vi "niRFUtil MASMT Get 1D CSG Type.vi"(1 "1D CSG Array in":csg[](array[numeric])) -> (0 "1D CSG Array out":csg[](array[numeric]))   [LabVIEW 2016, in "niRFUtil.lvlib"]
uses:
  niRFUtil.lvlib
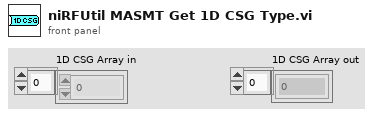
[diagram p1: front panel]
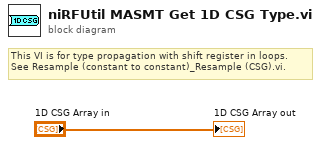
[diagram p0: block diagram]
diagram:
  # "This VI is for type propagation with shift register in loops.\nSee Resample (constant to constant)_Resample (CSG).vi."
  "1D CSG Array out" <- "1D CSG Array in"
